vi "svc_Copy Waveform Subset (Index).vi"(8 "error in (no error)":errorcluster, 9 "length (-1 = all)":i32=-1 min=-1 step=1, 10 "start index (0)":i32 step=1, 11 "waveform in":waveform(dbl)) -> (0 "error out":errorcluster, 1 "actual length":i32, 2 "actual start index":i32, 3 "waveform subset":waveform(dbl), 4 "end reached":bool)   [LabVIEW 2017]
doc: "Returns a portion of the waveform of the <B>start index</B> and <B>length</B> values. When you wire a waveform to this VI, the waveform automatically resizes to display <B>start index</B> inputs for the waveform."
uses:
  <vilib>/addons/_NISVFA/_Shared subVIs/Common/svc_Coerce Index and Length.vi
  <vilib>/addons/_NISVFA/_Shared subVIs/Common/svc_Conditional Merge Error.vi
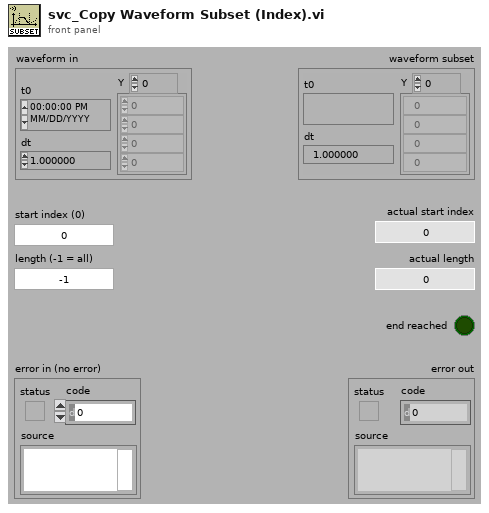
[diagram p1: front panel]
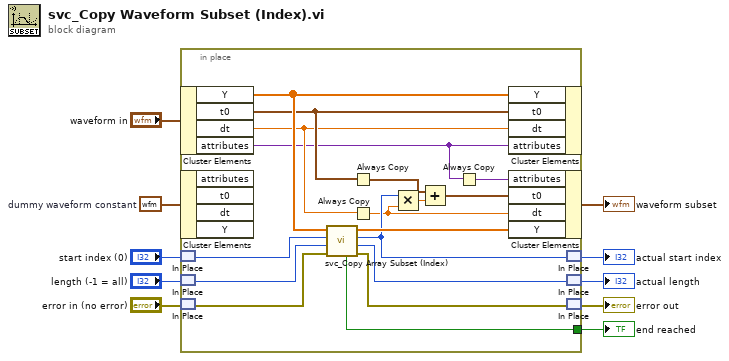
[diagram p0: block diagram]
diagram:
  w1 = waveform(dbl) {"t0"=timestamp(0 s since 1904-01-01), "dt"=1.0, "Y"=[]}  # dummy waveform constant
  n1 = in-place {
    in-place-border: [w20] -> w7
    n2 = in-place-cluster #1("waveform in") -> ("Y"=w17:dbl[], "t0"=w16:timestamp, "dt"=w14:dbl, "attributes"=w12:variant)
    n3 = in-place-cluster #2(w1) -> ()  [unwired: 4 out]
    n4 = in-place-match #3("start index (0)") -> (w25:i32)
    n5 = in-place-match #4("length (-1 = all)") -> (w24:i32)
    n6 = in-place-match #5("error in (no error)") -> (w19:errorcluster)
    n7 = call <vilib>:"svc_Copy Array Subset (Index).vi"("error in (no error)"=w19, "length (-1 = all)"=w24, "start index (0)"=w25, "Y"=w17) -> ("error out"=w18:errorcluster, "actual length"=w22:i32, "actual start index"=w21:i32, "Y subset"=w23:dbl[], "end reached"=w20:bool)  [unwired: 3 in]
    n8 = Always Copy(1:w16) -> (0:w15:timestamp)
    n9 = Always Copy(1:w14) -> (0:w13:dbl)
    n10 = Multiply(x=w21, y=w13) -> (x*y=w27:dbl)
    n11 = Add(x=w15, y=w27) -> (x+y=w26:timestamp)
    n12 = Always Copy(1:w12) -> (0:w11:variant)
    n13 = in-place-cluster #1("Y"=w17, "t0"=w16, "dt"=w14, "attributes"=w12) -> ()  [unwired: 1 out]
    n14 = in-place-cluster #2("attributes"=w11, "t0"=w26, "dt"=w13, "Y"=w23) -> (→"waveform subset":waveform(dbl))
    n15 = in-place-match #3(w21) -> (→"actual start index":i32)
    n16 = in-place-match #4(w22) -> (→"actual length":i32)
    n17 = in-place-match #5(w18) -> (→"error out":errorcluster)
  }
  "end reached" <- w7
